vi "Get Environment Variable.vi"(7 "Target (Process)":T1 items=["Process", "User", "Machine"], 8 "Error In":errorcluster, 11 "Name":string) -> (0 "Error Out":errorcluster, 3 "Value":string)   [LabVIEW 2023, in "SLL Environment Variable.lvlib"]
doc: "Get <B>Value</B> of environment variable from target environment."
uses:
  SLL Environment Variable.lvlib
  _Typedef/Target Environment Enum.ctl
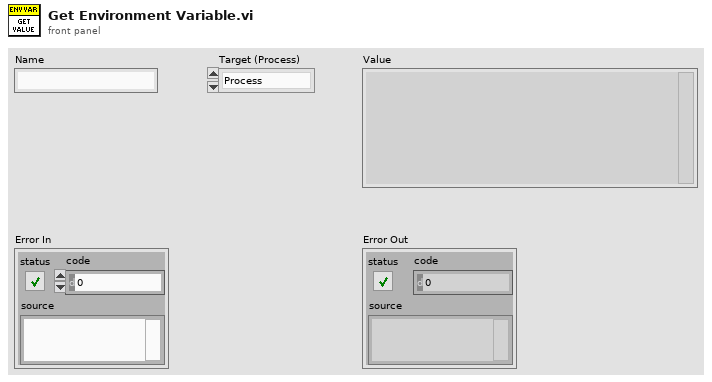
[diagram p1: front panel]
types:
  T1 = typedef "SLL Environment Variable.lvlib/Target Environment Enum.ctl" = i32
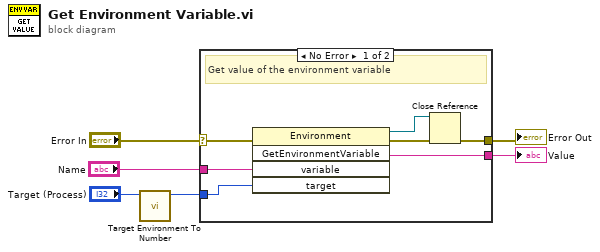
[diagram p0: block diagram]
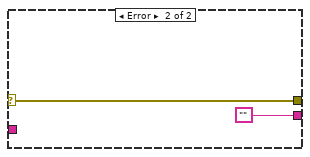
[diagram p2: hidden frame]
diagram:
  n1 = call "Target Environment To Number.vi"("Target (Process)"="Target (Process)") -> ("Number"=w1:i32)  [unwired: 10 in]
  n2 = case shown="No Error" "Error In" {
    selector: "Error In" -> [w13 w15]
    tunnel: "Name" -> [w12 _]
    tunnel: [w10 ""] -> w4
    tunnel: [w9 w15] -> w3
    tunnel: w1 -> [w7 _]
    frame No Error {
      # "Get value of the environment variable"
      n3 = invoke class="Environment" method="GetEnvironmentVariable"(error in=w13, "variable"=w12, "target"=w7) -> (reference out=w8:refnum<k24>, error out=w11:errorcluster, "GetEnvironmentVariable"=w10:string)  [unwired: 2 in, 2 out]
      n4 = Close Reference(reference=w8, error in (no error)=w11) -> (error out=w9:errorcluster)
    }
    frame Error {
    }
  }
  "Error Out" <- w3
  "Value" <- w4
